vi "Contour Line_Decide Height Vector.vi"(10 "number of heights":i32, 11 "Z":dbl[][](array[numeric])) -> (3 "Height Vector":dbl[](array[numeric]))   [LabVIEW 2020, in "NI_AAL_Geometry.lvlib"]
uses:
  <vilib>/Analysis/NI_AAL_Geometry.lvlib
  <vilib>/Analysis/NI_AALBase.lvlib
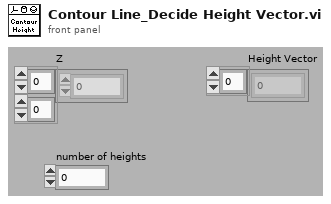
[diagram p1: front panel]
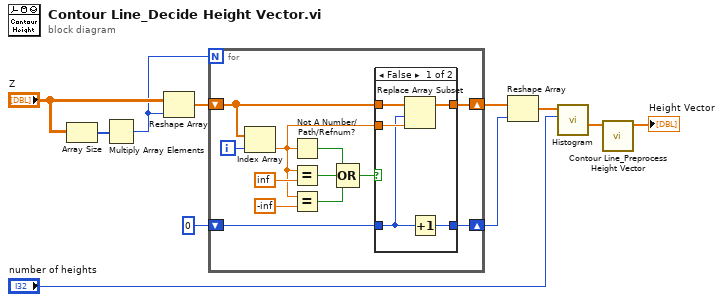
[diagram p0: block diagram]
diagram:
  n1 = Array Size(array="Z") -> (size(s)=w10:i32[])
  n2 = Multiply Array Elements(1:w10) -> (0:w9:i32)
  n3 = Reshape Array("Z", w9) -> (w8:dbl[])
  n4 = for {
    N: w9 -> [_]
    shift-right: [w16] -> w5
    shift-left: w8 -> [w17]
    shift-right: [w14] -> w6
    shift-left: 0 -> [w13]
    i -> [w12]
    n5 = Index Array(array=w17, index=w12) -> (element=w15:dbl)
    n6 = Not A Number/Path/Refnum?(number/path/refnum=w15) -> (NaN/Path/Refnum?=w20:bool)
    n7 = Equal?(x=w15, y=inf) -> (x = y?=w21:bool)
    n8 = Equal?(x=w15, y=-inf) -> (x = y?=w19:bool)
    n9 = Compound Arithmetic op=OR(w20, w21, w19) -> (w18:bool)
    n10 = case shown="False" w18 {
      tunnel: w17 -> [w28 w30]
      tunnel: [w27 w30] -> w16
      tunnel: w15 -> [w26 _]
      tunnel: w13 -> [w25 w29]
      tunnel: [w24 w29] -> w14
      frame False {
        n11 = Replace Array Subset(array=w28, new element=w26, index=w25) -> (w27:dbl[])
        n12 = Increment(x=w25) -> (x+1=w24:i32)
      }
      frame True {
      }
    }
  }
  n13 = Reshape Array(w5, w6) -> (w4:dbl[])
  n14 = call <vilib>:"Histogram.vi"("intervals"="number of heights", "X"=w4) -> ("X Values"=w3:dbl[])  [unwired: 9 out]
  n15 = call <vilib>:"Contour Line_Preprocess Height Vector.vi"("Height Vector In"=w3) -> ("Height Vector Out"=→"Height Vector":dbl[])  [unwired: 10 out]
